vi "GlobalFlash.vi"() -> ()   [LabVIEW 2017]
panel:
  out "AlarmArmed":bool
  out "AlarmTriggered":bool
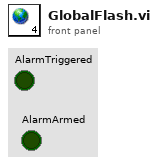
[diagram p1: front panel]
diagram:
